vi "escritura de archivo.vi"(10 "Array in":string[][](array[string]), 11 "Numeric":dbl) -> ()   [LabVIEW 2015]
uses:
  <vilib>/Utility/file.llb/Write Delimited Spreadsheet (string).vi
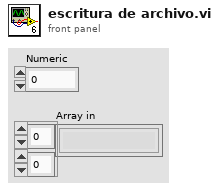
[diagram p1: front panel]
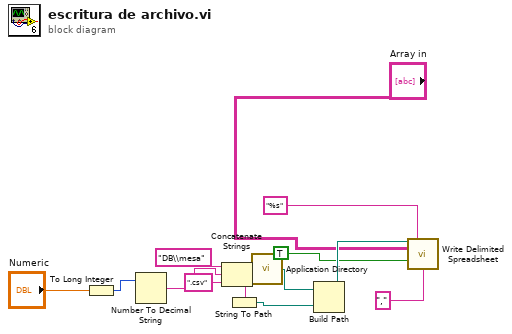
[diagram p0: block diagram]
diagram:
  n1 = To Long Integer(number="Numeric") -> (32bit integer=w9:i32)
  n2 = Number To Decimal String(number=w9) -> (decimal integer string=w7:string)  [unwired: 1 in]
  n3 = Concatenate Strings("DB\\mesa", w7, ".csv" ("string")) -> (w10:string)
  n4 = String To Path(string=w10) -> (path=w11:path)
  n5 = call <vilib>:"Application Directory.vi"() -> ("Application Directory"=w13:path)
  n6 = Build Path(base path=w13, name or relative path=w11) -> (appended path=w12:path)
  n7 = call-poly <vilib>:"Write Delimited Spreadsheet.vi"("file path (dialog if empty)"=w12, "format (%s)"="%s", "2D data"="Array in", "append to file? (F)"=TRUE, "delimiter (\\t)"="," ("delimiter (\\t)")) -> ()  [unwired: 9 in, 2 out]
